vi "Analisis de Amplitud y FFT.vi"() -> ()   [LabVIEW 2019]
uses:
  <instrlib>/niScope/Acquire/niScope Read WDT.vi
  <vilib>/express/express analysis/Spectral/Block/exnSpectralBlock spectral measurements power poly.vi
  <vilib>/express/express analysis/Spectral/Block/exnSpectralBlock spectral measurements power WFM.vi
  <vilib>/express/express analysis/Spectral/XNode/ExpressSpectralMeasurementsBlockNode.xnode
panel:
  out "Waveform Graph":cluster{"f0":dbl, "df":dbl, "magnitude":dbl[]}(graph)
  in  "resource name":refnum<k15>
  out "Amplitud":dbl
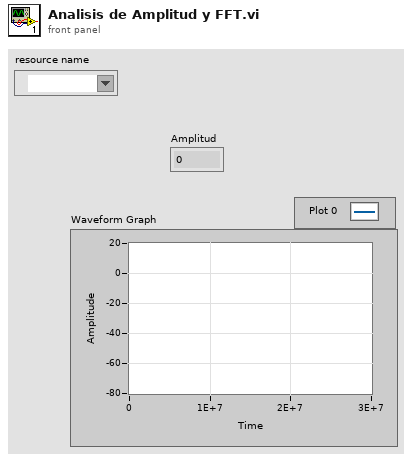
[diagram p1: front panel]
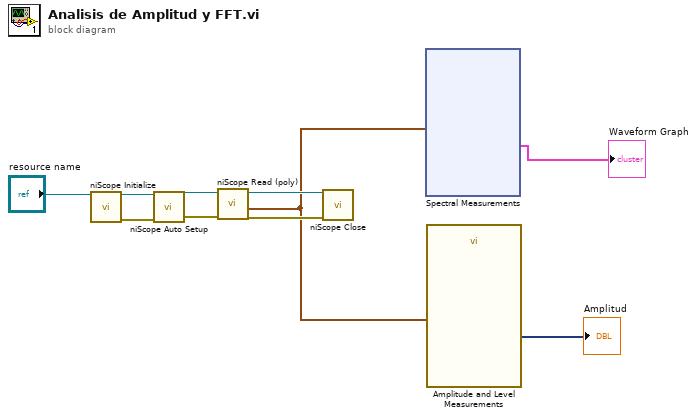
[diagram p0: block diagram]
diagram:
  n1 = call <instrlib>:"niScope Initialize.vi"("resource name"="resource name") -> ("instrument handle"=w10:refnum<k15>, "error out"=w9:errorcluster)  [unwired: 13 in]
  n2 = call <instrlib>:"niScope Auto Setup.vi"("instrument handle"=w10, "error in"=w9) -> ("instrument handle out"=w8:refnum<k15>, "error out"=w7:errorcluster)  [unwired: 12 in]
  n3 = call-poly <instrlib>:"niScope Read (poly).vi"("error in"=w7, "instrument handle"=w8) -> ("error out"=w5:errorcluster, "wfm"=w3:waveform(dbl), "instrument handle out"=w6:refnum<k15>)  [unwired: 6 in, 1 out]
  n4 = call <instrlib>:"niScope Close.vi"("instrument handle"=w6, "error in"=w5) -> ()  [unwired: 13 in, 1 out]
  n5 = xnode "Spectral Measurements"("Signals"=w3) -> ("Power Spectrum"=→"Waveform Graph":cluster{"f0":dbl, "df":dbl, "magnitude":dbl[]})  [unwired: 1 in, 1 out]
  n6 = call "Amplitude and Level Measurements"("Signals"=w3) -> ("Peak to Peak"=→"Amplitud":dynamicdata)  [unwired: 13 in, 1 out]
